vi "Wavelength to strain.vi"(11 "Wavelength":dbl[](array[numeric])) -> (3 "Strain":dbl[](array[numeric]))   [LabVIEW 2015]
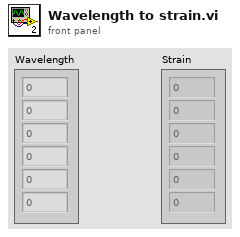
[diagram p1: front panel]
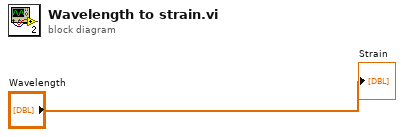
[diagram p0: block diagram]
diagram:
  "Strain" <- "Wavelength"
